vi "I3252_Edit_Temperature.vi"(1 "Temp. String":string) -> (0 "Temp. (°C)":dbl)   [LabVIEW 2013]
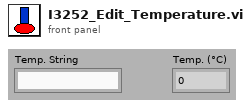
[diagram p1: front panel]
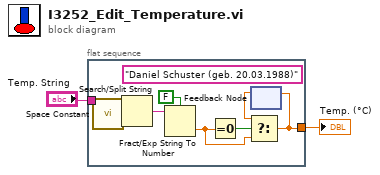
[diagram p0: block diagram]
diagram:
  (unwired) "Daniel Schuster (geb. 20.03.1988)"
  n1 = flat-sequence {
    tunnel: "Temp. String" -> [w4]
    tunnel: [w3] -> w1
    frame #0 {
      n2 = call <vilib>:"Space Constant.vi"() -> ("String"=w8:string)
      n3 = Search/Split String(string=w4, search string/char (-)=w8) -> (match + rest of string=w9:string)  [unwired: 1 in, 2 out]
      n4 = Fract/Exp String To Number(use system decimal point (T)=FALSE, string=w9) -> (number=w6:dbl)  [unwired: 2 in, 1 out]
      n5 = Equal To 0?(x=w6) -> (x = 0?=w7:bool)
      n6 = feedback #1() -> (w5:dbl)  [unwired: 1 in]
      n7 = Select(t=w5, s=w7, f=w6) -> (s? t:f=w3:dbl)
      n8 = feedback-in #1(w3) -> ()
    }
  }
  "Temp. (°C)" <- w1
